vi "Insert BLOB data.vi"(5 "Data In (Variants)":variant[](array[variant]), 6 "error in":errorcluster, 7 "Recordset Parameters":cluster{"CursorType":T1, "LockType":T2}={"CursorType"=0, "LockType"=1} {"CursorType" items=["adOpenUnspecified"=-1, "adOpenForwardOnly"=0, "adOpenKeyset"=1, "adOpenDynamic"=2, "adOpenStatic"=3]; "LockType" items=["adLockUnspecified"=-1, "adLockReadOnly"=1, "adLockPessimistic"=2, "adLockOptimistic"=3, "adLockBatchOptimistic"=4]}, 8 "BLOB Recordset definition Script":string, 9 "Connection In":refnum<k7>) -> (0 "error out":errorcluster, 3 "Connection Out":refnum<k7>)   [LabVIEW 2022 SP3, in "hse-db-ado.lvlib" / "ADO-DB-Driver.lvlib"]
doc: "Insert BLOB data\n\n____\nHAMPEL SOFTWARE ENGINEERING v1.4.0 (2023-12-19 09:52)"
uses:
  ADO-DB-Driver.lvlib
  _typedefs/CursorType.ctl
  _typedefs/LockType.ctl
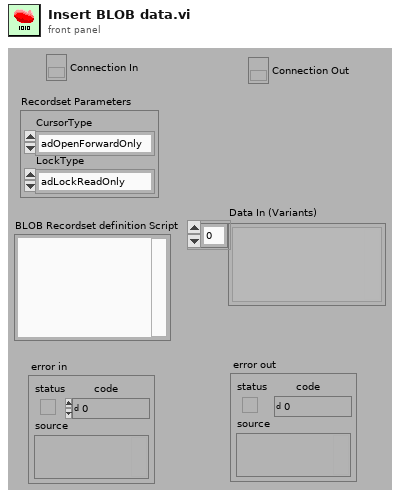
[diagram p1: front panel]
types:
  T1 = typedef "hse-db-ado.lvlib/ADO-DB-Driver.lvlib/CursorType.ctl" = i32
  T2 = typedef "hse-db-ado.lvlib/ADO-DB-Driver.lvlib/LockType.ctl" = i32
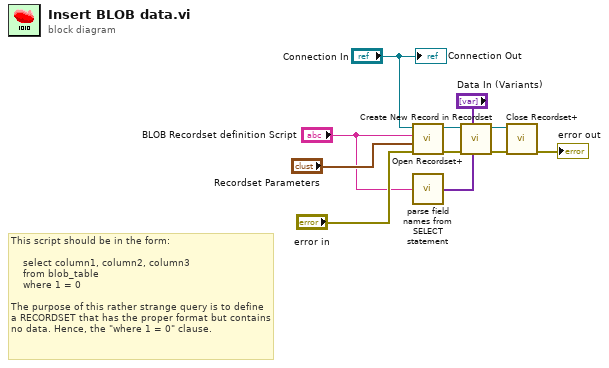
[diagram p0: block diagram]
diagram:
  # "This script should be in the form:\n\n    select column1, column2, column3\n    from blob_table\n    where 1 = 0\n\nThe purpose of this rather strange query is to define a RECORDSET that has the proper format but contains no data. Hence, the \"where 1 = 0\" clause."
  n1 = call "Open Recordset+.vi"("error in (no error)"="error in", "Recordset Parameters"="Recordset Parameters", "Source"="BLOB Recordset definition Script", "Connection"="Connection In") -> ("error out"=w7:errorcluster, "Recordset"=w8:refnum<k7>)  [unwired: 6 in]
  n2 = call "parse field names from SELECT statement.vi"("Select String"="BLOB Recordset definition Script") -> ("variant(field names)"=w5:variant[])
  n3 = call "Create New Record in Recordset.vi"("Field Names"=w5, "Field Values"="Data In (Variants)", "error in (no error)"=w7, "Recordset"=w8) -> ("error out"=w9:errorcluster, "Recordset Out"=w10:refnum<k7>)  [unwired: 4 in]
  n4 = call "Close Recordset+.vi"("error in"=w9, "Recordset"=w10) -> ("error out"=→"error out":errorcluster)  [unwired: 9 in]
  "Connection Out" <- "Connection In"
